vi "Update Test Run Result.vi"(8 "error in (no error)":errorcluster, 10 "Duration [ms]":u32, 11 "Single Thread Test Runner in":refnum<class "Parallell Test Runner.lvclass">) -> (0 "error out":errorcluster)   [LabVIEW 2020, in "Parallell Test Runner.lvclass"]
uses:
  Parallell Test Runner.lvclass
  Core/Result/Result.ctl
  Core/Result/Status.ctl
  Core/Result/Type.ctl
  Parallell Test Runner.lvclass/Parallell Test Runner.ctl
  Result Observer/Result Observer.lvclass
  Core/Result/Result.lvlib
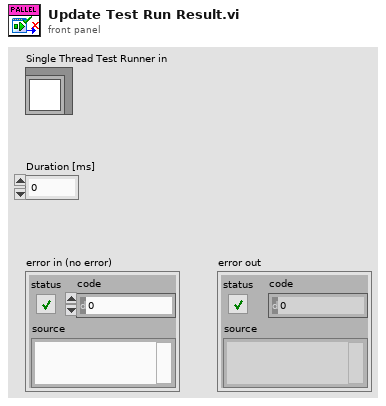
[diagram p1: front panel]
types:
  T1 = typedef "Result.lvlib/Result.ctl" = cluster{"Name":string, "Description":string, "Status":T2, "Result Type":T3, "Execution Time":dbl, "Data":cluster{"Expected":variant, "Actual":variant, "Delta":variant}}
  T2 = typedef "Result.lvlib/Status.ctl" = enum16{"", "Passed", "Failed", "Error", "Skipped", "Setup Error", "Broken", "Teardown Error"}
  T3 = typedef "Result.lvlib/Type.ctl" = enum16{"Test Case", "Test Suite", "Test Run", "Pass", "Fail", "Skip", "Pass if", "Fail if", "Pass if Error", "Fail if Error", "Pass if Equal", "Fail if Equal"}
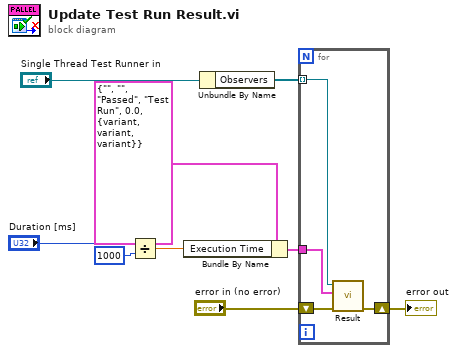
[diagram p0: block diagram]
diagram:
  n1 = Divide(x="Duration [ms]", y=u32 1000) -> (x/y=w1:dbl)
  n2 = Bundle By Name(cluster=T1 {"Name"="", "Description"="", "Status"=enum."Passed", "Result Type"=enum."Test Run", "Execution Time"=0.0, "Data"={"Expected"=variant, "Actual"=variant, "Delta"=variant}} ("Result"), "Execution Time"=w1) -> (w5:T1)
  n3 = Unbundle By Name("Single Thread Test Runner in") -> ("Observers"=w3:refnum<class "Result Observer.lvclass">[])
  n4 = for {
    tunnel: w3 -> [w13] mode=indexing
    tunnel: w5 -> [w12]
    shift-right: [w10] -> w9
    shift-left: "error in (no error)" -> [w11]
    n5 = call-dynamic "Result.vi"("error in (no error)"=w11, "Result"=w12, "Result Observer In"=w13) -> ("error out"=w10:errorcluster)  [unwired: 8 in]
  }
  "error out" <- w9
